vi "USB cmd send, no ACK.vi"(6 "Error In":errorcluster, 7 "4 byte config str":string, 8 "Cmd":T1="P", 9 "VISA resource name in":refnum<visa-resource-name>) -> (0 "Error out":errorcluster, 3 "VISA resource name out":refnum<visa-resource-name>)   [LabVIEW 2015]
uses:
  Ctls/Cmd str.ctl
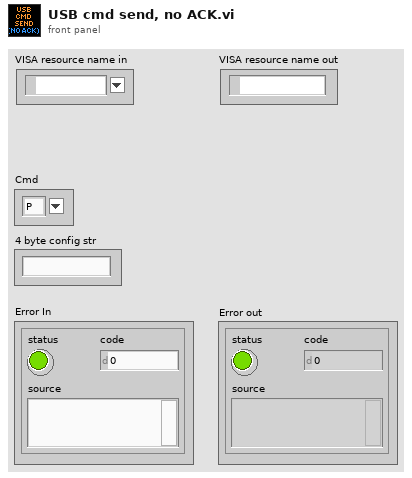
[diagram p1: front panel]
types:
  T1 = typedef "Cmd str.ctl" = string
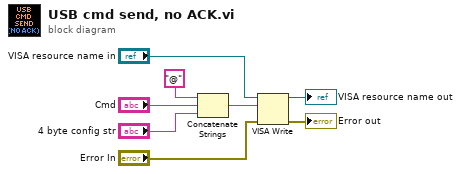
[diagram p0: block diagram]
diagram:
  n1 = Concatenate Strings("@" ("string"), "Cmd", "4 byte config str") -> (w3:string)
  n2 = VISA Write(VISA resource name="VISA resource name in", write buffer=w3, error in (no error)="Error In") -> (VISA resource name out=→"VISA resource name out":refnum<visa-resource-name>, error out=→"Error out":errorcluster)  [unwired: 1 out]
